vi "CompareLastHWI_NIcard.vi"(9 "Last NI card HWI":T1, 10 "NI card HWI":T1) -> (2 "change?":bool)   [LabVIEW 2013]
doc: "Compare all NI Card hardware info (Terminal Info, AO and AI channels, AO and DO array) and return \"change?\" boolean if anything changes."
uses:
  Utils/Unequal_safe/Unequal_Safe_2dBOOL.vi
  Utils/Unequal_safe/Unequal_Safe_2dDBL.vi
  Utils/Unequal_safe/Unequal_Safe_AnalogChArray.vi
panel:
  out "Term. Info Diff?":bool
  out "AI Ch Diff?":bool
  out "AO Ch Diff?":bool
  out "AO Diff?":bool
  out "DO Diff?":bool
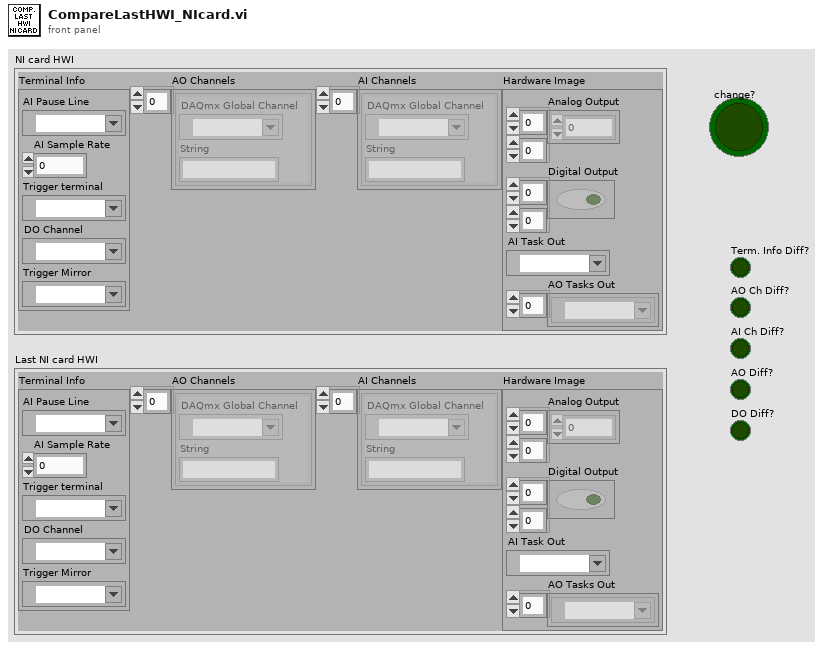
[diagram p1: front panel]
types:
  T1 = cluster{"Terminal Info":cluster{"AI Pause Line":tag, "AI Sample Rate":dbl, "Trigger terminal":tag, "DO Channel":refnum<k21>, "Trigger Mirror":tag}, "AO Channels":cluster{"DAQmx Global Channel":refnum<k21>, "String":string}[], "AI Channels":cluster{"DAQmx Global Channel":refnum<k21>, "String":string}[], "Hardware Image":cluster{"Analog Output ":dbl[][], "Digital Output":bool[][], "AI Task Out":refnum<k21>, "AO Tasks Out":refnum<k21>[]}}
  T2 = cluster{"AI Pause Line":tag, "AI Sample Rate":dbl, "Trigger terminal":tag, "DO Channel":refnum<k21>, "Trigger Mirror":tag}
  T3 = cluster{"DAQmx Global Channel":refnum<k21>, "String":string}[]
  T4 = cluster{"AI Pause Line":bool, "AI Sample Rate":bool, "Trigger terminal":bool, "DO Channel":bool, "Trigger Mirror":bool}
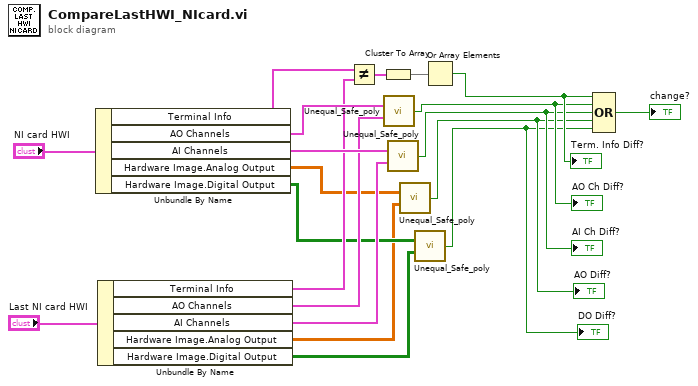
[diagram p0: block diagram]
diagram:
  n1 = Unbundle By Name("NI card HWI") -> ("Terminal Info"=w19:T2, "AO Channels"=w16:T3, "AI Channels"=w15:T3, "Hardware Image.Analog Output"=w9:dbl[][], "Hardware Image.Digital Output"=w10:bool[][])
  n2 = Unbundle By Name("Last NI card HWI") -> ("Terminal Info"=w13:T2, "AO Channels"=w12:T3, "AI Channels"=w11:T3, "Hardware Image.Analog Output"=w8:dbl[][], "Hardware Image.Digital Output"=w7:bool[][])
  n3 = Not Equal?(x=w19, y=w13) -> (x != y?=w18:T4)
  n4 = Cluster To Array(cluster=w18) -> (array=w17:bool[])
  n5 = call-poly "Unequal_Safe_poly.vi"("Analog Channels x"=w16, "Analog Channels y"=w12) -> ("Diff?"=w4:bool)  [unwired: 12 in, 1 out]
  "AO Ch Diff?" <- w4
  n6 = call-poly "Unequal_Safe_poly.vi"("Analog Channels x"=w15, "Analog Channels y"=w11) -> ("Diff?"=w3:bool)  [unwired: 12 in, 1 out]
  "AI Ch Diff?" <- w3
  n7 = call-poly "Unequal_Safe_poly.vi"("x"=w9, "y"=w8) -> ("Diff?"=w2:bool)  [unwired: 12 in, 1 out]
  "AO Diff?" <- w2
  n8 = call-poly "Unequal_Safe_poly.vi"("x"=w10, "y"=w7) -> ("Diff?"=w1:bool)  [unwired: 12 in, 1 out]
  "DO Diff?" <- w1
  n9 = Or Array Elements(Boolean array=w17) -> (logical OR=w5:bool)
  "Term. Info Diff?" <- w5
  n10 = Compound Arithmetic op=OR(w5, w4, w3, w2, w1) -> (→"change?":bool)
